vi "INI.LoadParameters.vi"(8 "error in (no error)":errorcluster caption="错误输入（无错误）", 9 "Specification_In":string[][](table), 10 "Command":enum16{"Load", "Save"}(ring), 11 "INI_File":path) -> (0 "error out":errorcluster, 1 "Specification_Out":string[][](table), 3 "ok?":bool)   [LabVIEW 2012, in "Lib_UEL.ATE.lvlib" / "Lib_App.lvlib"]
uses:
  Lib_App.lvlib
  <vilib>/Utility/config.llb/Read Key (String).vi
  <vilib>/Utility/config.llb/Write Key (String).vi
  <vilib>/Utility/config.llb/NI_LVConfig.lvlib
panel:
  # "要求：\n- 自动加载配置文件的规格参数到表格\n- 配置文件格式统一：项目,单位,参考值,生产下限,生产上限,QA下限,QA上限\n- 如果没有QA数据, 则QA与生产一致.\n- 如果没有生产数据, 表示是普通参数, 不是规格参数.\n\n注意\n- 只适用与参数, 端口,路径等的设置, 还是需要独立操作.\n- 配置文件分段: [sys]: 独立配置, [para]:参数配置"
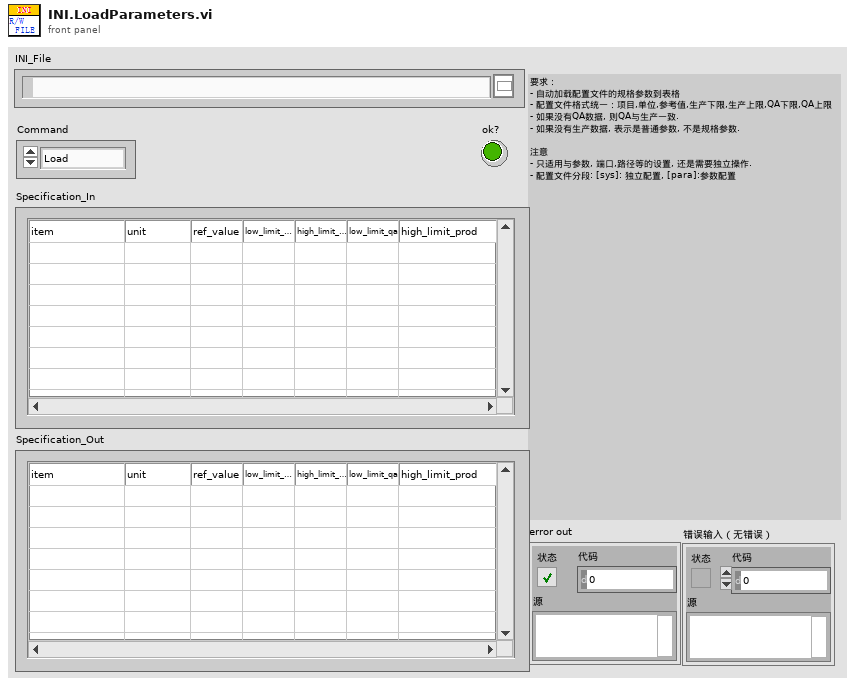
[diagram p1: front panel]
types:
  T1 = typedef "NI_LVConfig.lvlib/Config Data RefNum.ctl" = refnum<k1>
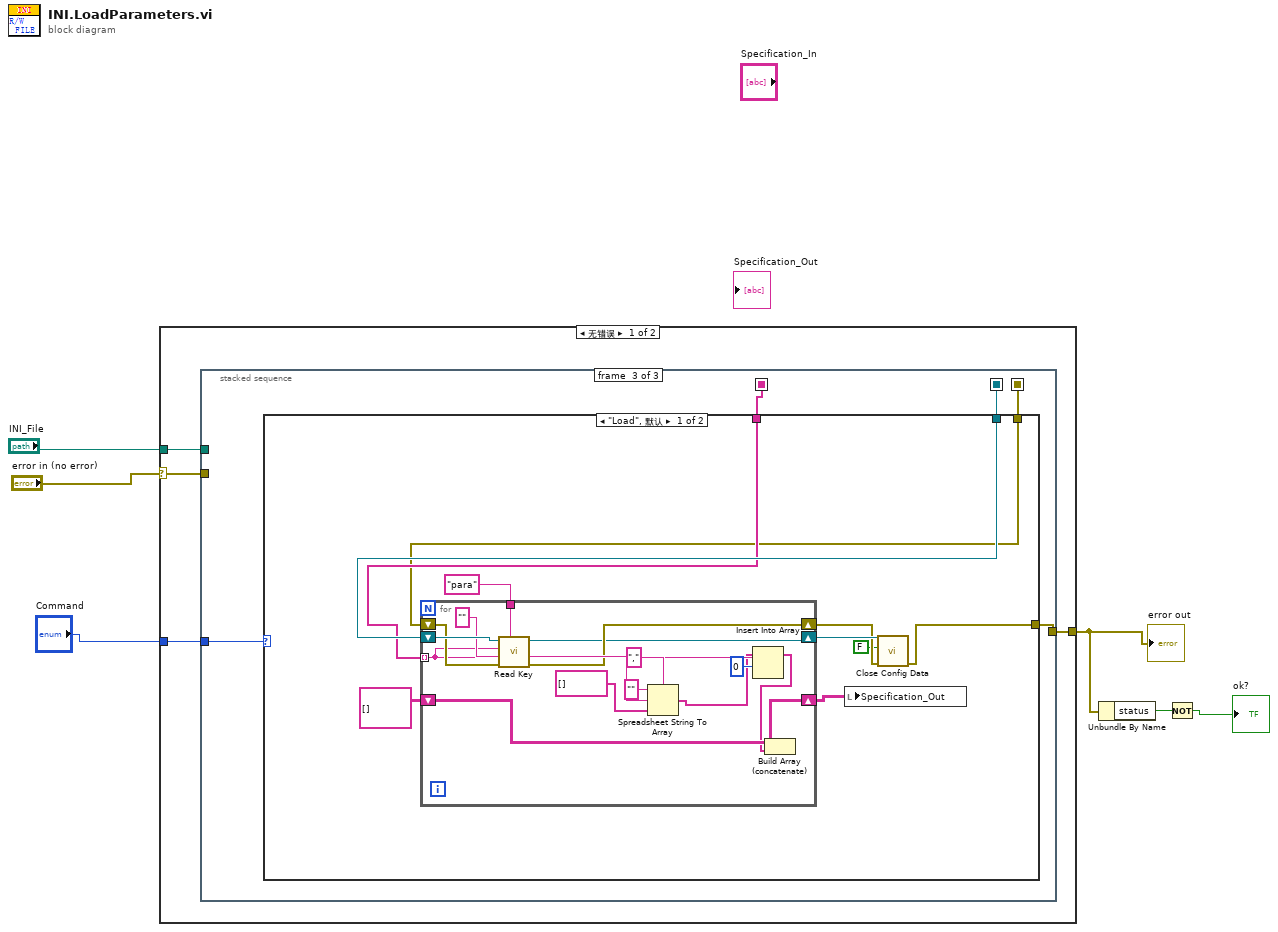
[diagram p0: block diagram]
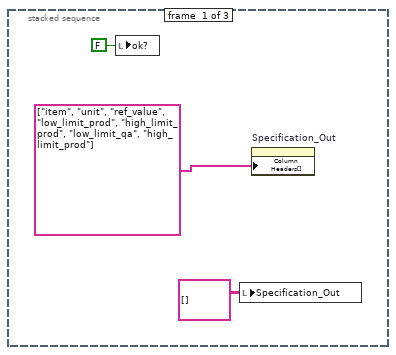
[diagram p2: hidden frame]
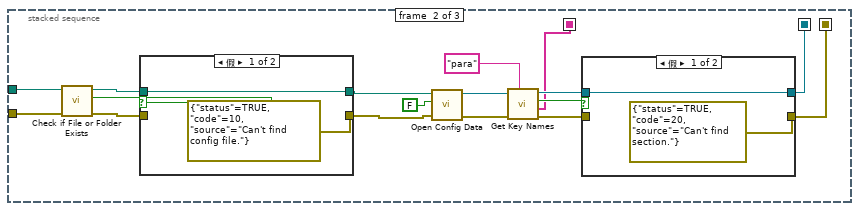
[diagram p3: hidden frame]
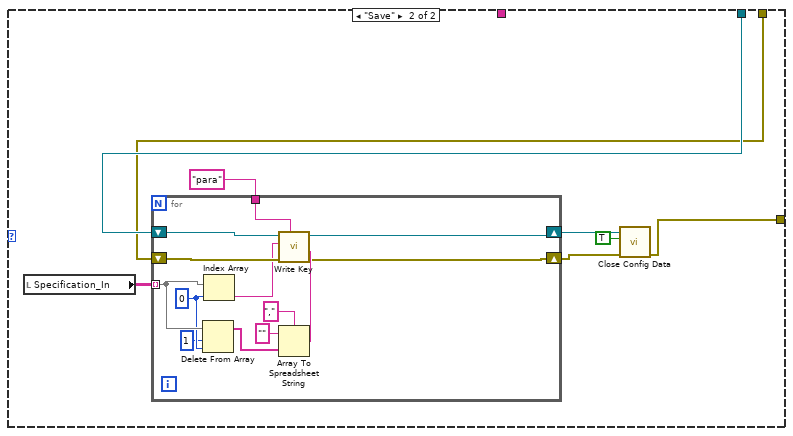
[diagram p6: hidden frame]
diagram:
  n1 = case shown="无错误" "error in (no error)" {
    selector: "error in (no error)" -> [w9 w91]
    tunnel: "INI_File" -> [w10 _]
    tunnel: [w8 w91] -> w3
    tunnel: "Command" -> [w7 _]
    frame No Error {
      n2 = stacked-sequence {
        seq-local: [_ w16 _] -> [_ _ w41]
        seq-local: [_ w15 _] -> [_ _ w42]
        seq-local: [_ w14 _] -> [_ _ w40]
        tunnel: w10 -> [_ w26 _]
        tunnel: w9 -> [_ w25 _]
        tunnel: [_ _ w43] -> w8
        tunnel: w7 -> [_ _ w39]
        frame #0 {
          n3 = local write "ok?"(FALSE ("ok?")) -> ()
          n4 = local write "Specification_Out"(string[][] [] ("Specification_Out")) -> ()
          n5 = property on="Specification_Out" class="Tbl (严格)"("Column Headers[]"=string[] ["item", "unit", "ref_value", "low_limit_prod", "high_limit_prod", "low_limit_qa", "high_limit_prod"] ("列首字符串[]")) -> ()  [unwired: 2 in, 2 out]
        }
        frame #1 {
          n6 = call <vilib>:"Check if File or Folder Exists.vi"("error in (no error)"=w25, "path"=w26) -> ("error out"=w28:errorcluster, "file or folder exists?"=w29:bool, "dup path"=w27:path)  [unwired: 7 in]
          n7 = case shown="假" w29 {
            tunnel: w28 -> [_ w37]
            tunnel: w27 -> [w36 w38]
            tunnel: [w36 w38] -> w24
            tunnel: [errorcluster {"status"=TRUE, "code"=10, "source"="Can't find config file."} ("error out") w37] -> w23
            frame False {
            }
            frame True {
            }
          }
          n8 = call <vilib>:"Open Config Data.vi"("error in (no error)"=w23, "create file if necessary (T)"=FALSE ("create file if necessary? (T)"), "configuration file path"=w24) -> ("error out"=w21:errorcluster, "refnum"=w20:T1)  [unwired: 6 in, 1 out]
          n9 = call <vilib>:"Get Key Names.vi"("section"="para", "error in (no error)"=w21, "refnum"=w20) -> ("error out"=w17:errorcluster, "key names"=w16:string[], "section exists?"=w19:bool, "refnum out"=w18:T1)  [unwired: 5 in]
          n10 = case shown="假" w19 {
            tunnel: w17 -> [_ w33]
            tunnel: w18 -> [w32 w34]
            tunnel: [w32 w34] -> w15
            tunnel: [errorcluster {"status"=TRUE, "code"=20, "source"="Can't find section."} ("error out") w33] -> w14
            frame False {
            }
            frame True {
            }
          }
        }
        frame #2 {
          n11 = case shown="\"Load\", 默认" w39 {
            tunnel: [w45 w71] -> w43
            tunnel: w42 -> [w50 w76]
            tunnel: w41 -> [w49 _]
            tunnel: w40 -> [w48 w75]
            frame "Load", Default {
              n12 = for {
                tunnel: "para" ("section") -> [w69]
                tunnel: w49 -> [w56] mode=indexing
                shift-right: [w61] -> w51
                shift-left: string[][] [] -> [w62]
                shift-right: [w60] -> w46
                shift-left: w48 -> [w67]
                shift-right: [w55] -> w47
                shift-left: w50 -> [w68]
                n13 = call-poly <vilib>:"Read Key.vi"("section"=w69, "error in (no error)"=w67, "default value"="" ("section"), "key"=w56, "refnum"=w68) -> ("error out"=w60:errorcluster, "value"=w63:string, "refnum out"=w55:T1)  [unwired: 3 in, 1 out]
                n14 = Spreadsheet String To Array(delimiter (Tab)="," ("分隔符(Tab)"), format string="" ("格式字符串"), spreadsheet string=w63, array type (2D Dbl)=string[] [] ("数组类型(2D Dbl)")) -> (array=w54:string[])
                n15 = Insert Into Array(array=w54, index=0 ("索引"), new element=w56) -> (w58:string[])
                n16 = Build Array (concatenate)(w62, w58) -> (w61:string[][])
              }
              n17 = local write "Specification_Out"(w51) -> ()
              n18 = call <vilib>:"Close Config Data.vi"("error in (no error)"=w46, "write file if changed (T)"=FALSE, "refnum"=w47) -> ("error out"=w45:errorcluster)  [unwired: 7 in, 1 out]
            }
            frame "Save" {
              n19 = local read "Specification_In"() -> (w74:string[][])
              n20 = for {
                tunnel: "para" ("section") -> [w90]
                shift-right: [w85] -> w72
                shift-left: w75 -> [w88]
                tunnel: w74 -> [w81] mode=indexing
                shift-right: [w84] -> w73
                shift-left: w76 -> [w89]
                w80 = 0 ("索引")
                n21 = Delete From Array(array=w81, length=1 ("长度"), index=w80) -> (array with subset deleted=w78:string[])  [unwired: 1 out]
                n22 = Index Array(array=w81, index=w80) -> (element=w82:string)
                n23 = Array To Spreadsheet String(delimiter (Tab)="," ("分隔符(Tab)"), array=w78, 3:"" ("格式字符串")) -> (spreadsheet string=w86:string)
                n24 = call-poly <vilib>:"Write Key.vi"("section"=w90, "error in (no error)"=w88, "value"=w86, "key"=w82, "refnum"=w89) -> ("error out"=w85:errorcluster, "refnum out"=w84:T1)  [unwired: 4 in, 1 out]
              }
              n25 = call <vilib>:"Close Config Data.vi"("error in (no error)"=w72, "write file if changed (T)"=TRUE, "refnum"=w73) -> ("error out"=w71:errorcluster)  [unwired: 7 in, 1 out]
            }
          }
        }
      }
    }
    frame Error {
    }
  }
  "error out" <- w3
  n26 = Unbundle By Name(w3) -> ("status"=w2:bool)
  n27 = Not(x=w2) -> (.not. x?=→"ok?":bool)
